vi "Reentrant Parallel SMU Meas (SubVI).vi"(8 "error in (no error)":errorcluster, 9 "current level":dbl, 10 "Channel List":string, 11 "IVI Refnum in":refnum<k15>) -> (0 "error out":errorcluster, 3 "Numeric":dbl)   [LabVIEW 2013]
uses:
  <instrlib>/niDCPower/nidcpower.llb/niDCPower Wait For Event - Event.ctl
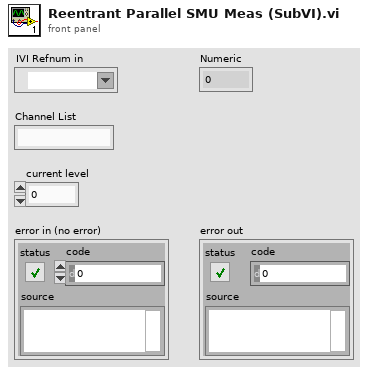
[diagram p1: front panel]
types:
  T1 = typedef "niDCPower Wait For Event - Event.ctl" = i32
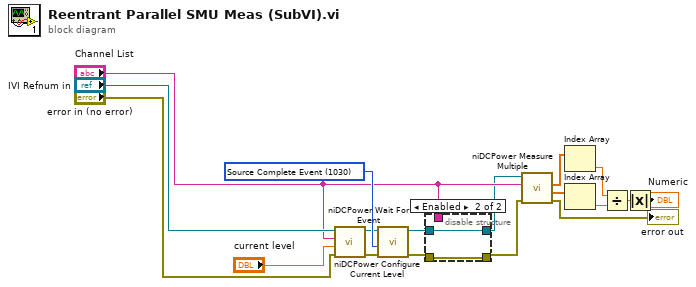
[diagram p0: block diagram]
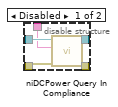
[diagram p2: hidden frame]
diagram:
  w15 = T1 1030 items=["Source Complete Event"=1030, "Measure Complete Event"=1031, "Sequence Iteration Complete Event"=1032, "Sequence Engine Done Event"=1033, "Pulse Complete Event"=1051, "Ready For Pulse Trigger Event"=1052] ("event")
  n1 = call <instrlib>:"niDCPower Configure Current Level.vi"("error in (no error)"="error in (no error)", "current level"="current level", "channel name"="Channel List", "instrument handle"="IVI Refnum in") -> ("error out"=w5:errorcluster, "instrument handle out"=w6:refnum<k15>)  [unwired: 6 in]
  n2 = call <instrlib>:"niDCPower Wait For Event.vi"("error in (no error)"=w5, "event"=w15, "instrument handle"=w6) -> ("error out"=w1:errorcluster, "instrument handle out"=w2:refnum<k15>)  [unwired: 7 in]
  n3 = disable-structure shown="Enabled" {
    disable-tunnel: w1 -> [w23 w25]
    disable-tunnel: w2 -> [w22 w24]
    disable-tunnel: [w21 w24] -> w3
    disable-tunnel: [w20 w25] -> w4
    disable-tunnel: "Channel List" -> [w19 _]
    frame Disabled {
      n4 = call <instrlib>:"niDCPower Query In Compliance.vi"("error in (no error)"=w23, "channel name"=w19, "instrument handle"=w22) -> ("error out"=w20:errorcluster, "instrument handle out"=w21:refnum<k15>)  [unwired: 6 in, 1 out]
    }
    frame Enabled {
    }
  }
  n5 = call <instrlib>:"niDCPower Measure Multiple.vi"("error in (no error)"=w4, "channel name"="Channel List", "instrument handle"=w3) -> ("error out"=→"error out":errorcluster, "current measurements"=w12:dbl[], "voltage measurements"=w11:dbl[])  [unwired: 5 in, 1 out]
  n6 = Index Array(array=w11) -> (element=w9:dbl)  [unwired: 1 in]
  n7 = Index Array(array=w12) -> (element=w10:dbl)  [unwired: 1 in]
  n8 = Divide(x=w9, y=w10) -> (x/y=w8:dbl)
  n9 = Absolute Value(x=w8) -> (abs(x)=→"Numeric":dbl)
